vi "Write white player.vi"(8 "error in (no error)":errorcluster, 10 "WhitePlayer":string, 11 "CS++GoBangClient in":refnum<class "CS++GoBangClient.lvclass">) -> (0 "error out":errorcluster, 3 "CS++GoBangClient out":refnum<class "CS++GoBangClient.lvclass">)   [LabVIEW 2013, in "GoBang.lvlib" / "CS++GoBangClient.lvclass"]
uses:
  CS++GoBangClient.lvclass
  CS++GoBangClient.lvclass/CS++GoBangClient.ctl
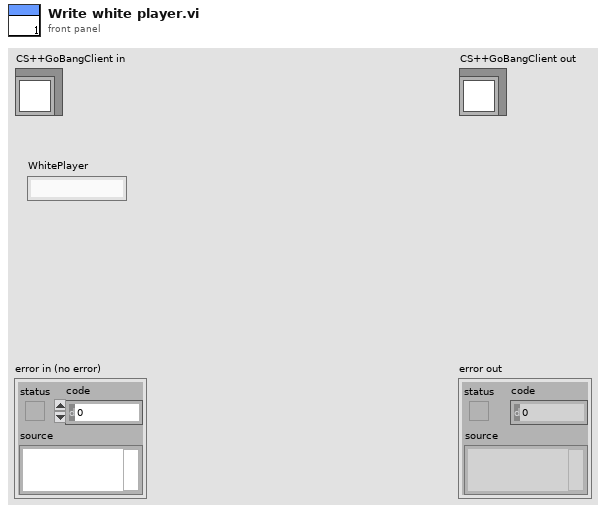
[diagram p1: front panel]
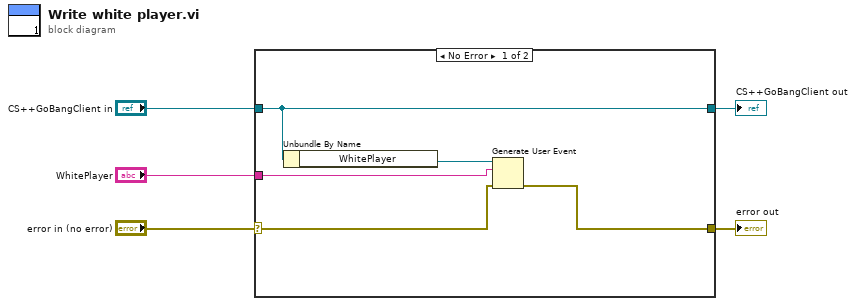
[diagram p0: block diagram]
diagram:
  n1 = case shown="No Error" "error in (no error)" {
    selector: "error in (no error)" -> [w7 w12]
    tunnel: [w6 w12] -> w4
    tunnel: [w10 w11] -> w2
    tunnel: "CS++GoBangClient in" -> [w10 w11]
    tunnel: "WhitePlayer" -> [w8 _]
    frame No Error {
      n2 = Unbundle By Name(w10) -> ("WhitePlayer"=w9:refnum<user-event>)
      n3 = Generate User Event(user event=w9, event data cluster=w8, error in=w7) -> (error out=w6:errorcluster)  [unwired: 1 in, 1 out]
    }
    frame Error {
    }
  }
  "error out" <- w4
  "CS++GoBangClient out" <- w2
